vi "DELETE ObtainNotifiers.vi"(8 "error in (no error)":errorcluster, 11 "DAQmx":refnum<class "DAQmx.lvclass">) -> (0 "error out":errorcluster, 3 "DAQmx out":refnum<class "DAQmx.lvclass">)   [LabVIEW 2019]
uses:
  DAQmx.lvclass
  typedefs/DAQ.Config.Timing.Sampling--Cluster.ctl
  typedefs/DAQ.Config.Timing.Fs Mode--enum.ctl
  typedefs/DAQ.Config.Timing--Cluster.ctl
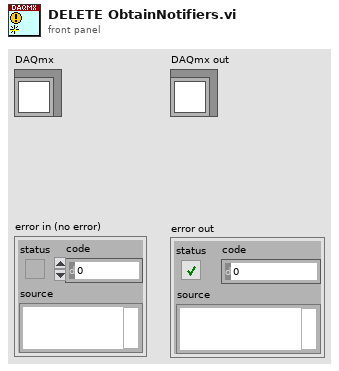
[diagram p1: front panel]
types:
  T1 = typedef "DAQmx.lvclass/DAQ.Config.Timing--Cluster.ctl" = cluster{"Sampling":T2, "sample mode":i32, "FsMode":T3, "Fs Multiplier":dbl, "Refresh Rate (Hz)":dbl, "Decimation.PreDSP":i32, "Decimation.PostDSP":i32, "Fs.Output":dbl}
  T2 = typedef "DAQmx.lvclass/DAQ.Config.Timing.Sampling--Cluster.ctl" = cluster{"Fs":dbl, "#s":i32}
  T3 = typedef "DAQmx.lvclass/DAQ.Config.Timing.Fs Mode--enum.ctl" = enum16{"Manual", "Auto Fs", "Max Fs"}
  T4 = typedef "DAQmx.lvclass/PrivateEvents--Cluster.ctl" = cluster{"State":refnum<user-event>, "AOconfig":refnum<user-event>, "AIconfig":refnum<user-event>, "Timing":refnum<user-event>}
  T5 = typedef "DAQmx.lvclass/DAQmx.States--enum.ctl" = enum16{"idle", "start", "stop", "calibrate", "auto", "exit"}
  T6 = typedef "DAQmx.lvclass/DAQ.Config.AO--Cluster--Array.ctl" = T7[]
  T7 = typedef "DAQmx.lvclass/DAQ.Config.AO--Cluster.ctl" = cluster{"Channels":tag, "Range":T8, "output terminal configuration":i32, "Type":T9}
  T8 = typedef "DAQmx.lvclass/DAQ.Config.AO.Range--enum.ctl" = enum16{"±0.1", "±1.0", "±10.0", ""}
  T9 = typedef "DAQmx.lvclass/DAQ.Config.Device Type--enum.ctl" = enum16{"None", "USB-4431", "PXI-446x"}
  T10 = typedef "DAQmx.lvclass/DAQ.Config.AI--Cluster--Array.ctl" = T11[]
  T11 = typedef "DAQmx.lvclass/DAQ.Config.AI--Cluster.ctl" = cluster{"Channels":tag, "Coupling":T12, "Range":T13, "input terminal configuration":i32, "Type":T9}
  T12 = typedef "DAQmx.lvclass/DAQ.Config.AI.Coupling--enum.ctl" = u16
  T13 = typedef "DAQmx.lvclass/DAQ.Config.AI.Range--enum.ctl" = enum16{"±0.316", "±1.00", "±3.16", "±10.0", "±31.6", "±42.4", ""}
  T14 = cluster{"setState":T5, "AOconfig":T6, "AIconfig":T10, "Timing":T1}
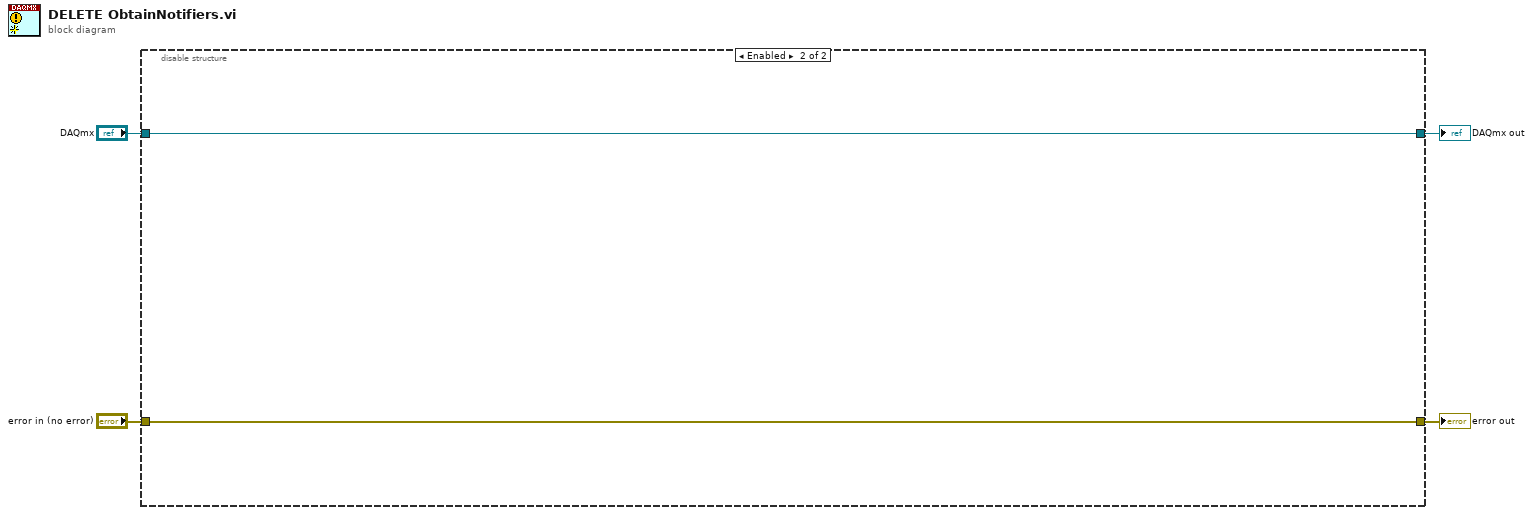
[diagram p0: block diagram]
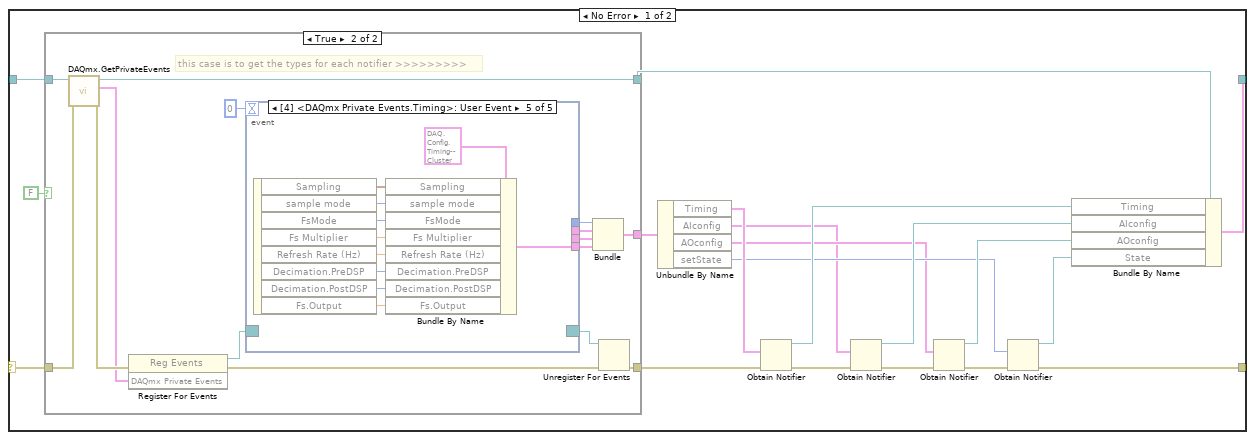
[diagram p3: hidden frame]
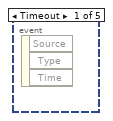
[diagram p5: hidden frame]
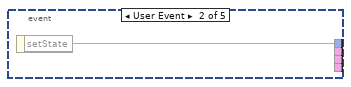
[diagram p6: hidden frame]
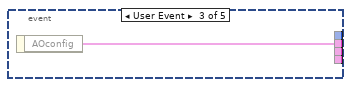
[diagram p7: hidden frame]
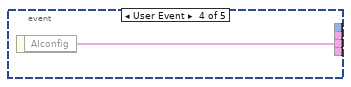
[diagram p8: hidden frame]
diagram:
  n1 = disable-structure shown="Enabled" {
    disable-tunnel: "DAQmx" -> [w8 w61]
    disable-tunnel: [w7 w61] -> w3
    disable-tunnel: "error in (no error)" -> [w6 w60]
    disable-tunnel: [w5 w60] -> w1
    frame Disabled {
      n2 = case shown="Error .." w6 {
        selector: w6 -> [w18 w59]
        tunnel: w8 -> [w26 w58]
        tunnel: [w24 w58] -> w7
        tunnel: [w16 w59] -> w5
        frame No Error {
          n3 = case shown="True" FALSE {
            tunnel: [_ w39] -> w27
            tunnel: w26 -> [w29 w38]
            tunnel: [w29 w34] -> w19
            tunnel: w18 -> [w28 w33]
            tunnel: [w28 w32] -> w13
            frame False {
            }
            frame True {
              # "this case is to get the types for each notifier >>>>>>>>>"
              n4 = call "DAQmx.GetPrivateEvents.vi"("error in (no error)"=w33, "DAQmx"=w38) -> ("error out"=w31:errorcluster, "DAQmx Private Events"=w30:T4, "DAQmx out"=w34:refnum<class "DAQmx.lvclass">)  [unwired: 7 in]
              n5 = register-events(error in=w31, w30) -> (reference out=w40:refnum<event-registration>, error out=w36:errorcluster)  [unwired: 1 in]
              n6 = event shown="[4] <DAQmx Private Events.Timing>: User Event" {
                selector: w40 -> [_ _ _ _ _]
                dyn-events: [_ _ _ _ _] -> w37
                timeout: 0 -> [_ _ _ _ _]
                tunnel: [_ w45 _ _ _] -> w44
                tunnel: [_ _ w46 _ _] -> w43
                tunnel: [_ _ _ w47 _] -> w42
                tunnel: [_ _ _ _ w56] -> w41
                event Timeout {
                  n7 = event-data() -> ()  [unwired: 1 in, 3 out]
                }
                event User Event {
                  n8 = event-data() -> ("setState"=w45:T5)  [unwired: 1 in]
                }
                event User Event {
                  n9 = event-data() -> ("AOconfig"=w46:T6)  [unwired: 1 in]
                }
                event User Event {
                  n10 = event-data() -> ("AIconfig"=w47:T10)  [unwired: 1 in]
                }
                event User Event {
                  n11 = event-data() -> ("Sampling"=w55:T2, "sample mode"=w54:i32, "FsMode"=w53:T3, "Fs Multiplier"=w52:dbl, "Refresh Rate (Hz)"=w51:dbl, "Decimation.PreDSP"=w50:i32, "Decimation.PostDSP"=w49:i32, "Fs.Output"=w48:dbl)  [unwired: 1 in]
                  n12 = Bundle By Name(cluster=T1 {"Sampling"={"Fs"=1000.0, "#s"=128}, "sample mode"=10123, "FsMode"=enum."Manual", "Fs Multiplier"=1.0, "Refresh Rate (Hz)"=10.0, "Decimation.PreDSP"=1, "Decimation.PostDSP"=1, "Fs.Output"=204789.0} ("Timing"), "Sampling"=w55, "sample mode"=w54, "FsMode"=w53, "Fs Multiplier"=w52, "Refresh Rate (Hz)"=w51, "Decimation.PreDSP"=w50, "Decimation.PostDSP"=w49, "Fs.Output"=w48) -> (w56:T1)
                }
              }
              n13 = Bundle("setState"=w44, "AOconfig"=w43, "AIconfig"=w42, "Timing"=w41) -> (w39:T14)  [unwired: 1 in]
              n14 = Unregister For Events(event registration refnum=w37, error in=w36) -> (error out=w32:errorcluster)
            }
          }
          n15 = Unbundle By Name(w27) -> ("Timing"=w25:T1, "AIconfig"=w10:T10, "AOconfig"=w11:T6, "setState"=w12:T5)
          n16 = Obtain Notifier(notification data type=w25, error in (no error)=w13) -> (notifier out=w23:refnum<notifier>, error out=w14:errorcluster)  [unwired: 2 in, 1 out]
          n17 = Obtain Notifier(notification data type=w10, error in (no error)=w14) -> (notifier out=w22:refnum<notifier>, error out=w15:errorcluster)  [unwired: 2 in, 1 out]
          n18 = Obtain Notifier(notification data type=w11, error in (no error)=w15) -> (notifier out=w21:refnum<notifier>, error out=w17:errorcluster)  [unwired: 2 in, 1 out]
          n19 = Obtain Notifier(notification data type=w12, error in (no error)=w17) -> (notifier out=w20:refnum<notifier>, error out=w16:errorcluster)  [unwired: 2 in, 1 out]
          n20 = Bundle By Name(cluster=w19, "Timing"=w23, "AIconfig"=w22, "AOconfig"=w21, "State"=w20) -> (w24:cluster{})
        }
        frame Error {
        }
      }
    }
    frame Enabled {
    }
  }
  "error out" <- w1
  "DAQmx out" <- w3
